vi "TW Post-Project-Copying Process - Stage 2.vi"(8 "error in":errorcluster, 10 "New Subname":string, 11 "Template Project Path":path) -> (0 "error out":errorcluster)   [LabVIEW 2021, in "Plugin Generator.lvlib"]
uses:
  Plugin Generator/Plugin Generator.lvlib
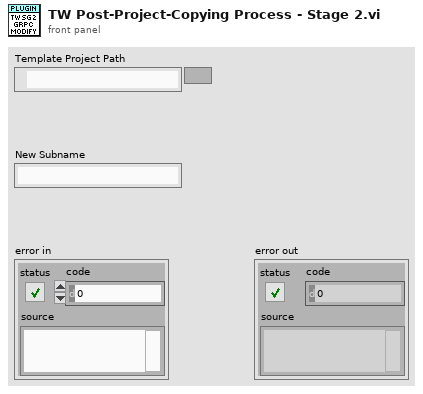
[diagram p1: front panel]
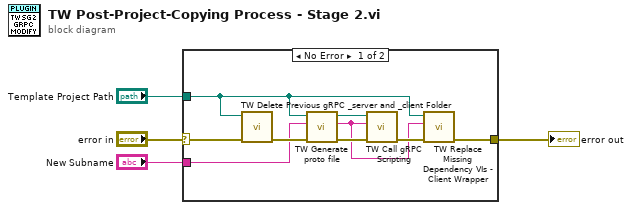
[diagram p0: block diagram]
diagram:
  n1 = case shown="No Error" "error in" {
    selector: "error in" -> [w7 w14]
    tunnel: [w12 w14] -> w4
    tunnel: "New Subname" -> [w6 _]
    tunnel: "Template Project Path" -> [w5 _]
    frame No Error {
      n2 = call "TW Delete Previous gRPC _server and _client Folder.vi"("error in"=w7, "Template Project Path"=w5) -> ("error out"=w8:errorcluster)  [unwired: 9 in]
      n3 = call "TW Generate proto file.vi"("error in"=w8, "New Subname"=w6, "Template Project Path"=w5) -> ("error out"=w11:errorcluster, "gRPC Service Name"=w9:string, "proto File Path"=w10:path)  [unwired: 6 in]
      n4 = call "TW Call gRPC Scripting.vi"("error in"=w11, "gRPC Service Name"=w9, "proto File Path"=w10) -> ("error out"=w13:errorcluster)  [unwired: 8 in]
      n5 = call "TW Replace Missing Dependency VIs - Client Wrapper.vi"("error in"=w13, "gRPC Service Name"=w9, "Template Project Path"=w5) -> ("error out"=w12:errorcluster)  [unwired: 8 in]
    }
    frame Error {
    }
  }
  "error out" <- w4
